vi "GetSingleAnalogInputVal.vi"(8 "error in (no error)":errorcluster, 10 "Pin number 0-7":dbl, 11 "SerialPortRef":T1) -> (0 "error out":errorcluster, 1 "Scaled Voltage":dbl, 2 "Raw Voltage":u32, 3 "SerialPortRef 2":T1)   [LabVIEW 2015]
uses:
  <vilib>/Rock Robotics/WPI/SerialPort/WPI_SerialPortRef.ctl
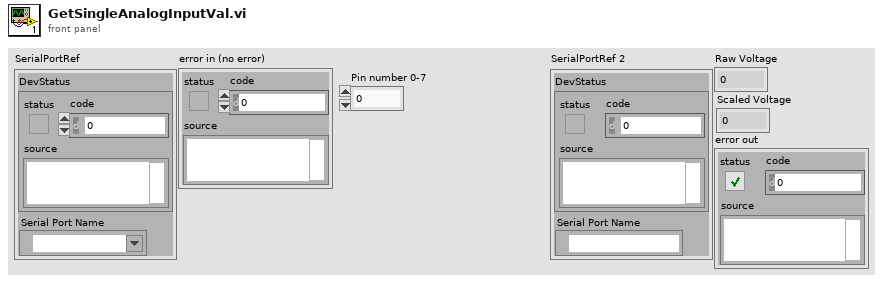
[diagram p1: front panel]
types:
  T1 = typedef "WPI_SerialPortRef.ctl" = cluster{"DevStatus":errorcluster, "Serial Port Name":refnum<visa-resource-name>}
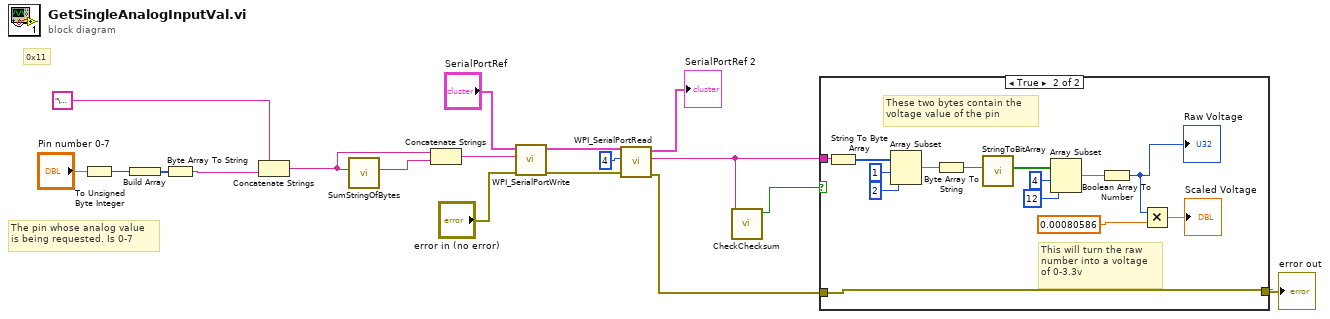
[diagram p0: block diagram]
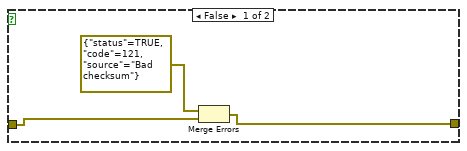
[diagram p2: hidden frame]
diagram:
  # "The pin whose analog value\nis being requested. Is 0-7"
  # "0x11"
  n1 = To Unsigned Byte Integer(number="Pin number 0-7") -> (unsigned 8bit integer=w4:u8)
  n2 = Build Array(w4) -> (w7:u8[])
  n3 = Byte Array To String(unsigned byte array=w7) -> (string=w2:string)
  n4 = Concatenate Strings("\u0011" ("Buffer"), w2) -> (w1:string)
  n5 = call "SumStringOfBytes.vi"("String Of Bytes"=w1) -> ("SumAsString"=w6:string)  [unwired: 10 in]
  n6 = Concatenate Strings(w1, w6) -> (w5:string)
  n7 = call <vilib>:"WPI_SerialPortWrite.vi"("error in (no error)"="error in (no error)", "Buffer"=w5, "SerialPortRef"="SerialPortRef") -> ("error out"=w14:errorcluster, "SerialPortRef"=w18:T1)  [unwired: 6 in, 1 out]
  n8 = call <vilib>:"WPI_SerialPortRead.vi"("error in (no error)"=w14, "Num Bytes to Read"=u32 4, "SerialPortRef"=w18) -> ("error out"=w9:errorcluster, "Buffer"=w12:string, "SerialPortRef"=→"SerialPortRef 2":T1)  [unwired: 6 in]
  n9 = call "CheckChecksum.vi"("String"=w12) -> ("x = y?"=w11:bool)  [unwired: 9 in, 1 out]
  n10 = case shown="True" w11 {
    tunnel: w12 -> [_ w23]
    tunnel: w9 -> [w21 w22]
    tunnel: [w19 w22] -> w10
    frame False {
      n11 = Merge Errors(errorcluster {"status"=TRUE, "code"=121, "source"="Bad checksum"} ("error in"), w21) -> (w19:errorcluster)
    }
    frame True {
      # "This will turn the raw \nnumber into a voltage \nof 0-3.3v"
      # "These two bytes contain the \nvoltage value of the pin"
      n12 = String To Byte Array(string=w23) -> (unsigned byte array=w35:u8[])
      n13 = Array Subset(array=w35, index=1, length=2) -> (w32:u8[])
      n14 = Byte Array To String(unsigned byte array=w32) -> (string=w31:string)
      n15 = call "StringToBitArray.vi"("string"=w31) -> ("Array"=w30:bool[])  [unwired: 10 in]
      n16 = Array Subset(array=w30, index=4, length=12) -> (w27:bool[])
      n17 = Boolean Array To Number(Boolean array=w27) -> (number=w26:u32)
      "Raw Voltage" <- w26
      n18 = Multiply(x=w26, y=0.00080586) -> (x*y=→"Scaled Voltage":dbl)
    }
  }
  "error out" <- w10
